vi "GetEvtSignal.vi"(8 "error in (no error)":errorcluster, 11 "RingdownEvtPlugin in":refnum<class "RingdownEvtPlugin.lvclass">) -> (0 "error out":errorcluster, 3 "RingdownEvtPlugin out":refnum<class "RingdownEvtPlugin.lvclass">)   [LabVIEW 2017, in "EventPlugins.lvlib" / "RingdownEvtPlugin.lvclass"]
uses:
  RingdownEvtPlugin.lvclass
  C:/dev/Work/PARTF/Modules/EventPlugins/EventPluginBaseClass/EventPluginBaseClass.lvclass
  EventPluginBaseClass/Accessors/Read EvtConfig.vi
  EventPluginBaseClass/Accessors/Read TimeArray.vi
  EventPluginBaseClass/Accessors/Read EvtParams.vi
  C37EvtPlugin/C37EvtPlugin.lvclass
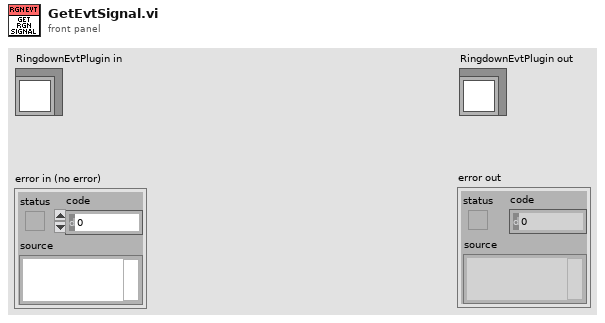
[diagram p1: front panel]
types:
  T1 = typedef "EventPlugins.lvlib/EventPluginBaseClass.lvclass/clEvtConfig.ctl" = cluster{"T0(UTC)":dbl, "F0":dbl, "Fs":i32, "FSamp":u32, "bPosSeq":bool}
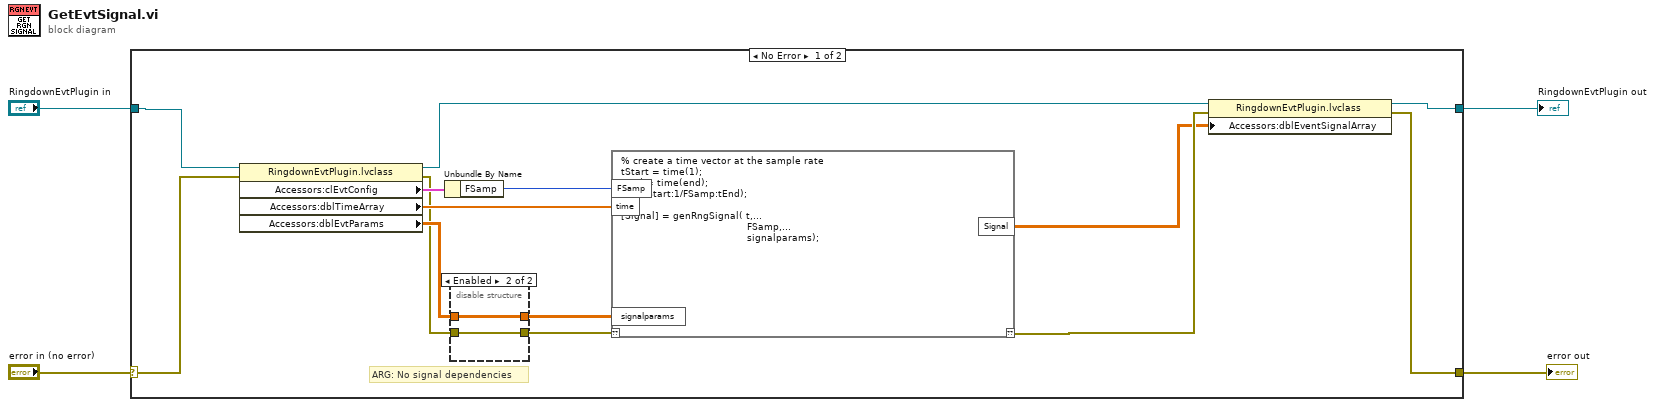
[diagram p0: block diagram]
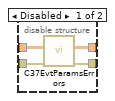
[diagram p2: hidden frame]
diagram:
  n1 = case shown="No Error" "error in (no error)" {
    selector: "error in (no error)" -> [w5 w26]
    tunnel: [w7 w26] -> w3
    tunnel: [w8 w25] -> w1
    tunnel: "RingdownEvtPlugin in" -> [w6 w25]
    frame No Error {
      # "ARG: No signal dependencies"
      n2 = property class="RingdownEvtPlugin.lvclass"(reference=w6, error in=w5) -> (reference out=w16:refnum<class "RingdownEvtPlugin.lvclass">, error out=w10:errorcluster, "Accessors:clEvtConfig"=w18:T1, "Accessors:dblTimeArray"=w14:dbl[], "Accessors:dblEvtParams"=w11:dbl[][])
      n3 = Unbundle By Name(w18) -> ("FSamp"=w17:u32)
      n4 = disable-structure shown="Enabled" {
        disable-tunnel: [w22 w23] -> w13
        disable-tunnel: [w21 w24] -> w12
        disable-tunnel: w11 -> [w20 w24]
        disable-tunnel: w10 -> [w19 w23]
        frame Disabled {
          n5 = call "C37EvtParamsErrors.vi"("error in (no error)"=w19, "dblSignalParams in"=w20) -> ("error out"=w22:errorcluster, "dblSignalParams out"=w21:dbl[][])  [unwired: 8 in]
        }
        frame Enabled {
        }
      }
      n6 = script code="% create a time vector at the sample rate\ntStart = time(1);\ntEnd = time(end);\nt = (tStart:1/FSamp:tEnd);\n\n[Signal] = genRngSignal( t,...\n                                          FSamp,...\n                                          signalparams);"("??"=w13, "FSamp"=w17, "time"=w14, "signalparams"=w12) -> ("??"=w15:errorcluster, "Signal"=w9:dbl[][])
      n7 = property class="RingdownEvtPlugin.lvclass"(reference=w16, error in=w15, "Accessors:dblEventSignalArray"=w9) -> (reference out=w8:refnum<class "RingdownEvtPlugin.lvclass">, error out=w7:errorcluster)
    }
    frame Error {
    }
  }
  "error out" <- w3
  "RingdownEvtPlugin out" <- w1
